vi "SwerveDrivePoseEst2_Update.vi"(6 "Time":dbl=-1.0 format="%33.4f", 9 "module Positions":T1[](array[typedef]) {"Angle"."SIN" format="%13.4f"; "Angle"."COS" format="%13.4f"; "Angle"."VALUE" format="%13.4f"}, 10 "GyroAngle":T2={"VALUE"=0.0, "COS"=1.0, "SIN"=0.0} {"SIN" format="%13.4f"; "COS" format="%13.4f"; "VALUE" format="%13.4f"}, 11 "in SwerveDrivePoseEstimate":T5={"M_Vision_K"=[], "m_nominal_dT"=0.0, "m_PrevTime_Sec"=0.0, "Pose_Buffer"={"TimeStamps"=[], "DataArray"=[], "Min_TimeStamp"=0.0, "Max_TimeStamp"=0.0, "ItemCount"=0, "MaxBufferTime"=0.0}, "Swerve_Drive_Kinematics"={"NumModules"=0, "InverseKinematics"=[], "ForwardKinematics"=[], "Modules"=[], "PrevCoR"={"X"=0.0, "Y"=0.0}, "SavedModuleStates"=[]}, "Swerve_Drive_Odom"={"POSE"={"TRANSLATION"={"X"=0.0, "Y"=0.0}, "ROTATION"={"VALUE"=0.0, "COS"=1.0, "SIN"=0.0}}, "GyroOffset"={"VALUE"=0.0, "COS"=1.0, "SIN"=0.0}, "PreviousAngle"={"VALUE"=0.0, "COS"=1.0, "SIN"=0.0}, "PrevModulePositions"=[], "NumModules"=0}, "M_Q"=[[0.0], [0.0], [0.0]], "NumModules"=-1} {"Swerve_Drive_Odom"."PrevModulePositions"."Angle"."SIN" format="%13.4f"; "Swerve_Drive_Odom"."PrevModulePositions"."Angle"."COS" format="%13.4f"; "Swerve_Drive_Odom"."PrevModulePositions"."Angle"."VALUE" format="%13.4f"; "Swerve_Drive_Odom"."PreviousAngle"."SIN" format="%13.4f"; "Swerve_Drive_Odom"."PreviousAngle"."COS" format="%13.4f"; "Swerve_Drive_Odom"."PreviousAngle"."VALUE" format="%13.4f"; "Swerve_Drive_Odom"."GyroOffset"."SIN" format="%13.4f"; "Swerve_Drive_Odom"."GyroOffset"."COS" format="%13.4f"; "Swerve_Drive_Odom"."GyroOffset"."VALUE" format="%13.4f"; "Swerve_Drive_Odom"."POSE"."ROTATION"."SIN" format="%13.4f"; "Swerve_Drive_Odom"."POSE"."ROTATION"."COS" format="%13.4f"; "Swerve_Drive_Odom"."POSE"."ROTATION"."VALUE" format="%13.4f"; "Swerve_Drive_Odom"."POSE"."TRANSLATION"."Y" format="%14.3f"; "Swerve_Drive_Odom"."POSE"."TRANSLATION"."X" format="%14.3f"; "Swerve_Drive_Kinematics"."SavedModuleStates"."Angle"."SIN" format="%13.4f"; "Swerve_Drive_Kinematics"."SavedModuleStates"."Angle"."COS" format="%13.4f"; "Swerve_Drive_Kinematics"."SavedModuleStates"."Angle"."VALUE" format="%13.4f"; "Swerve_Drive_Kinematics"."PrevCoR"."Y" format="%14.3f"; "Swerve_Drive_Kinematics"."PrevCoR"."X" format="%14.3f"; "Swerve_Drive_Kinematics"."Modules"."Y" format="%14.3f"; "Swerve_Drive_Kinematics"."Modules"."X" format="%14.3f"}) -> (0 "Error":bool, 2 "Estimated Pose":T3 {"ROTATION"."SIN" format="%13.4f"; "ROTATION"."COS" format="%13.4f"; "ROTATION"."VALUE" format="%13.4f"; "TRANSLATION"."Y" format="%14.3f"; "TRANSLATION"."X" format="%14.3f"}, 3 "Out SwerveDrivePoseEstimate":T5={"M_Vision_K"=[], "m_nominal_dT"=0.0, "m_PrevTime_Sec"=0.0, "Pose_Buffer"={"TimeStamps"=[], "DataArray"=[], "Min_TimeStamp"=0.0, "Max_TimeStamp"=0.0, "ItemCount"=0, "MaxBufferTime"=0.0}, "Swerve_Drive_Kinematics"={"NumModules"=0, "InverseKinematics"=[], "ForwardKinematics"=[], "Modules"=[], "PrevCoR"={"X"=0.0, "Y"=0.0}, "SavedModuleStates"=[]}, "Swerve_Drive_Odom"={"POSE"={"TRANSLATION"={"X"=0.0, "Y"=0.0}, "ROTATION"={"VALUE"=0.0, "COS"=1.0, "SIN"=0.0}}, "GyroOffset"={"VALUE"=0.0, "COS"=1.0, "SIN"=0.0}, "PreviousAngle"={"VALUE"=0.0, "COS"=1.0, "SIN"=0.0}, "PrevModulePositions"=[], "NumModules"=0}, "M_Q"=[[0.0], [0.0], [0.0]], "NumModules"=-1} {"Swerve_Drive_Odom"."PrevModulePositions"."Angle"."SIN" format="%13.4f"; "Swerve_Drive_Odom"."PrevModulePositions"."Angle"."COS" format="%13.4f"; "Swerve_Drive_Odom"."PrevModulePositions"."Angle"."VALUE" format="%13.4f"; "Swerve_Drive_Odom"."PreviousAngle"."SIN" format="%13.4f"; "Swerve_Drive_Odom"."PreviousAngle"."COS" format="%13.4f"; "Swerve_Drive_Odom"."PreviousAngle"."VALUE" format="%13.4f"; "Swerve_Drive_Odom"."GyroOffset"."SIN" format="%13.4f"; "Swerve_Drive_Odom"."GyroOffset"."COS" format="%13.4f"; "Swerve_Drive_Odom"."GyroOffset"."VALUE" format="%13.4f"; "Swerve_Drive_Odom"."POSE"."ROTATION"."SIN" format="%13.4f"; "Swerve_Drive_Odom"."POSE"."ROTATION"."COS" format="%13.4f"; "Swerve_Drive_Odom"."POSE"."ROTATION"."VALUE" format="%13.4f"; "Swerve_Drive_Odom"."POSE"."TRANSLATION"."Y" format="%14.3f"; "Swerve_Drive_Odom"."POSE"."TRANSLATION"."X" format="%14.3f"; "Swerve_Drive_Kinematics"."SavedModuleStates"."Angle"."SIN" format="%13.4f"; "Swerve_Drive_Kinematics"."SavedModuleStates"."Angle"."COS" format="%13.4f"; "Swerve_Drive_Kinematics"."SavedModuleStates"."Angle"."VALUE" format="%13.4f"; "Swerve_Drive_Kinematics"."PrevCoR"."Y" format="%14.3f"; "Swerve_Drive_Kinematics"."PrevCoR"."X" format="%14.3f"; "Swerve_Drive_Kinematics"."Modules"."Y" format="%14.3f"; "Swerve_Drive_Kinematics"."Modules"."X" format="%14.3f"})   [LabVIEW 2019, in "Trajectory_Library.lvlib"]
doc: "Updates the the robot odometry using only wheel encoder information. Note that this should be called every loop.\n\nInputs:\n - inSwerveDrivePoseEst -- system data cluster\n - gyroAngle -- The current gyro angle. (radians)\n - ModulePositions -- Array Module Position -- The current module positions (distance and angle)\n - currentTime -- Time at which this method was called, in seconds.\n\nOutputs:\n - outSwerveDrivePoseEst -- system data cluster\n - EstimatedPose -- The estimated pose of the robot in meters."
uses:
  Trajectory_Library.lvlib
  TypeDef/SWERVE_DRIVE_POSE_EST2.ctl
  <vilib>/Analysis/Matrix/Datatypes/RealMatrix.ctl
  TypeDef/TIME_INTERPOLATABLE_VARIANT.ctl
  TypeDef/SWERVE_DRIVE_KINEMATICS.ctl
  TypeDef/TRANSLATION2D.ctl
  TypeDef/SWERVE_DRIVE_MODULE_STATE.ctl
  TypeDef/ROTATION2D.ctl
  TypeDef/SWERVE_DRIVE_ODOMETRY.ctl
  TypeDef/POSE2D.ctl
  TypeDef/SWERVE_DRIVE_MODULE_POSITION.ctl
  Util_GetTime_U32.vi
  Util_GetTime_U64.vi
  <vilib>/Analysis/Matrix/NI_Matrix.lvlib
panel:
  # "<3, 1>"
  # "<3, 3>"
  # "<3, 1>"
  # "<3, 3>"
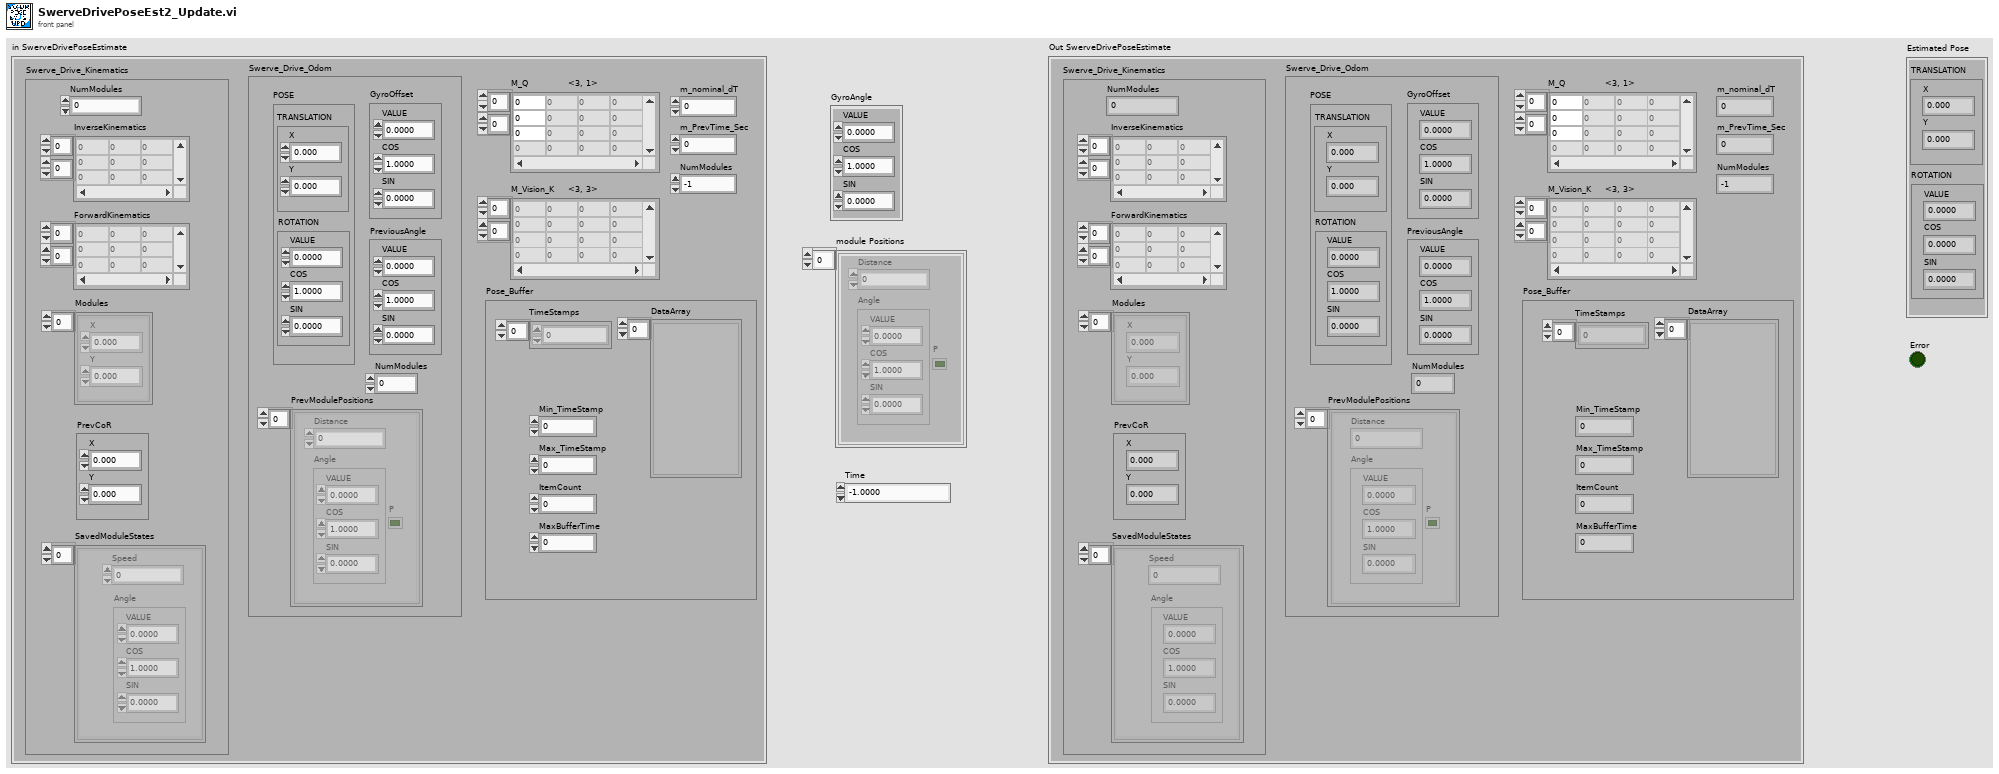
[diagram p1: front panel]
types:
  T1 = typedef "Trajectory_Library.lvlib/SWERVE_DRIVE_MODULE_POSITION.ctl" = cluster{"Distance":dbl, "Angle":T2, "P":bool}
  T2 = typedef "Trajectory_Library.lvlib/ROTATION2D.ctl" = cluster{"VALUE":dbl, "COS":dbl, "SIN":dbl}
  T3 = typedef "Trajectory_Library.lvlib/POSE2D.ctl" = cluster{"TRANSLATION":T4, "ROTATION":T2}
  T4 = typedef "Trajectory_Library.lvlib/TRANSLATION2D.ctl" = cluster{"X":dbl, "Y":dbl}
  T5 = typedef "Trajectory_Library.lvlib/SWERVE_DRIVE_POSE_EST2.ctl" = cluster{"M_Vision_K":T6, "m_nominal_dT":dbl, "m_PrevTime_Sec":dbl, "Pose_Buffer":T7, "Swerve_Drive_Kinematics":T8, "Swerve_Drive_Odom":T10, "M_Q":T6, "NumModules":i32}
  T6 = typedef "NI_Matrix.lvlib/RealMatrix.ctl" = dbl[][]
  T7 = typedef "Trajectory_Library.lvlib/TIME_INTERPOLATABLE_VARIANT.ctl" = cluster{"TimeStamps":dbl[], "DataArray":variant[], "Min_TimeStamp":dbl, "Max_TimeStamp":dbl, "ItemCount":i32, "MaxBufferTime":dbl}
  T8 = typedef "Trajectory_Library.lvlib/SWERVE_DRIVE_KINEMATICS.ctl" = cluster{"NumModules":i32, "InverseKinematics":T6, "ForwardKinematics":T6, "Modules":T4[], "PrevCoR":T4, "SavedModuleStates":T9[]}
  T9 = typedef "Trajectory_Library.lvlib/SWERVE_DRIVE_MODULE_STATE.ctl" = cluster{"Speed":dbl, "Angle":T2}
  T10 = typedef "Trajectory_Library.lvlib/SWERVE_DRIVE_ODOMETRY.ctl" = cluster{"POSE":T3, "GyroOffset":T2, "PreviousAngle":T2, "PrevModulePositions":T1[], "NumModules":i32}
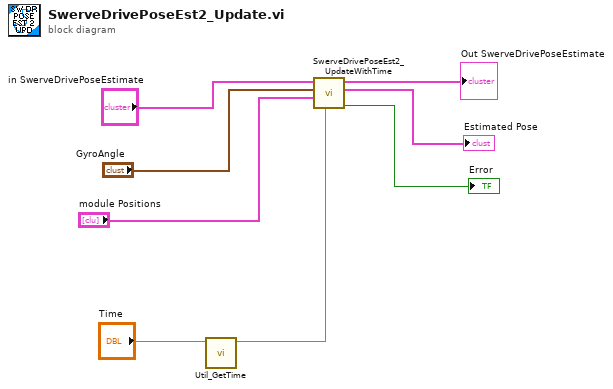
[diagram p0: block diagram]
diagram:
  n1 = call "Util_GetTime.vi"("Pass_Through_Time"="Time") -> ("FPGA_Time_Seconds"=w2:dbl)  [unwired: 8 in, 2 out]
  n2 = call "SwerveDrivePoseEst2_UpdateWithTime.vi"("CurrentTimeSeconds"=w2, "module Positions"="module Positions", "GyroAngle"="GyroAngle", "in SwerveDrivePoseEst2"="in SwerveDrivePoseEstimate") -> ("Error"=→"Error":bool, "Estimated Pose"=→"Estimated Pose":T3, "Out SwerveDrivePoseEst2"=→"Out SwerveDrivePoseEstimate":T5)  [unwired: 5 in]
